vi "SVA 4MV6 T030 CCE RRMA .vi"() -> ()   [LabVIEW 2020]
doc: "Ceballos Conde Emanuel Rodríguez Ramírez Miguel Ángel 4MV6 Sistemas de visión artificial 2022/1\neste vi permite obtener el borde en escala de grises de una imagen asi como la malla conformada por el angulo phi de la imagen"
uses:
  <vilib>/Math Plots/3D Math Plots/3D Mesh/3D Mesh XCtrl/3D Mesh.xctl
  <vilib>/Math Plots/3D Math Plots/3D Mesh/3D Mesh Datatype/Public/Plot Helper (Matrix).vi
  <vilib>/Math Plots/3D Math Plots/3D Mesh/3D Mesh Datatype/3D Mesh Datatype.lvclass
panel:
  in  "obtener borde":bool
  in  "stop":bool
  out "3D Mesh":refnum<class "3D Plot Datatype.lvclass">[](xcontrol)
  in  "amp borde":u8=1
  out "new picture 2":picture
  out "new picture":picture
  in  "sig":i32=2
  in  "T":i32=3
  in  "CAPA DE COLOR":T1(ring)=enum."RGB2GRAY MATLAB"
  in  "file":path
  # "Ceballos Conde Emanuel\nRodríguez Ramírez Miguel Ángel\n4MV6\nSistemas de visión artificial\n2022/1"
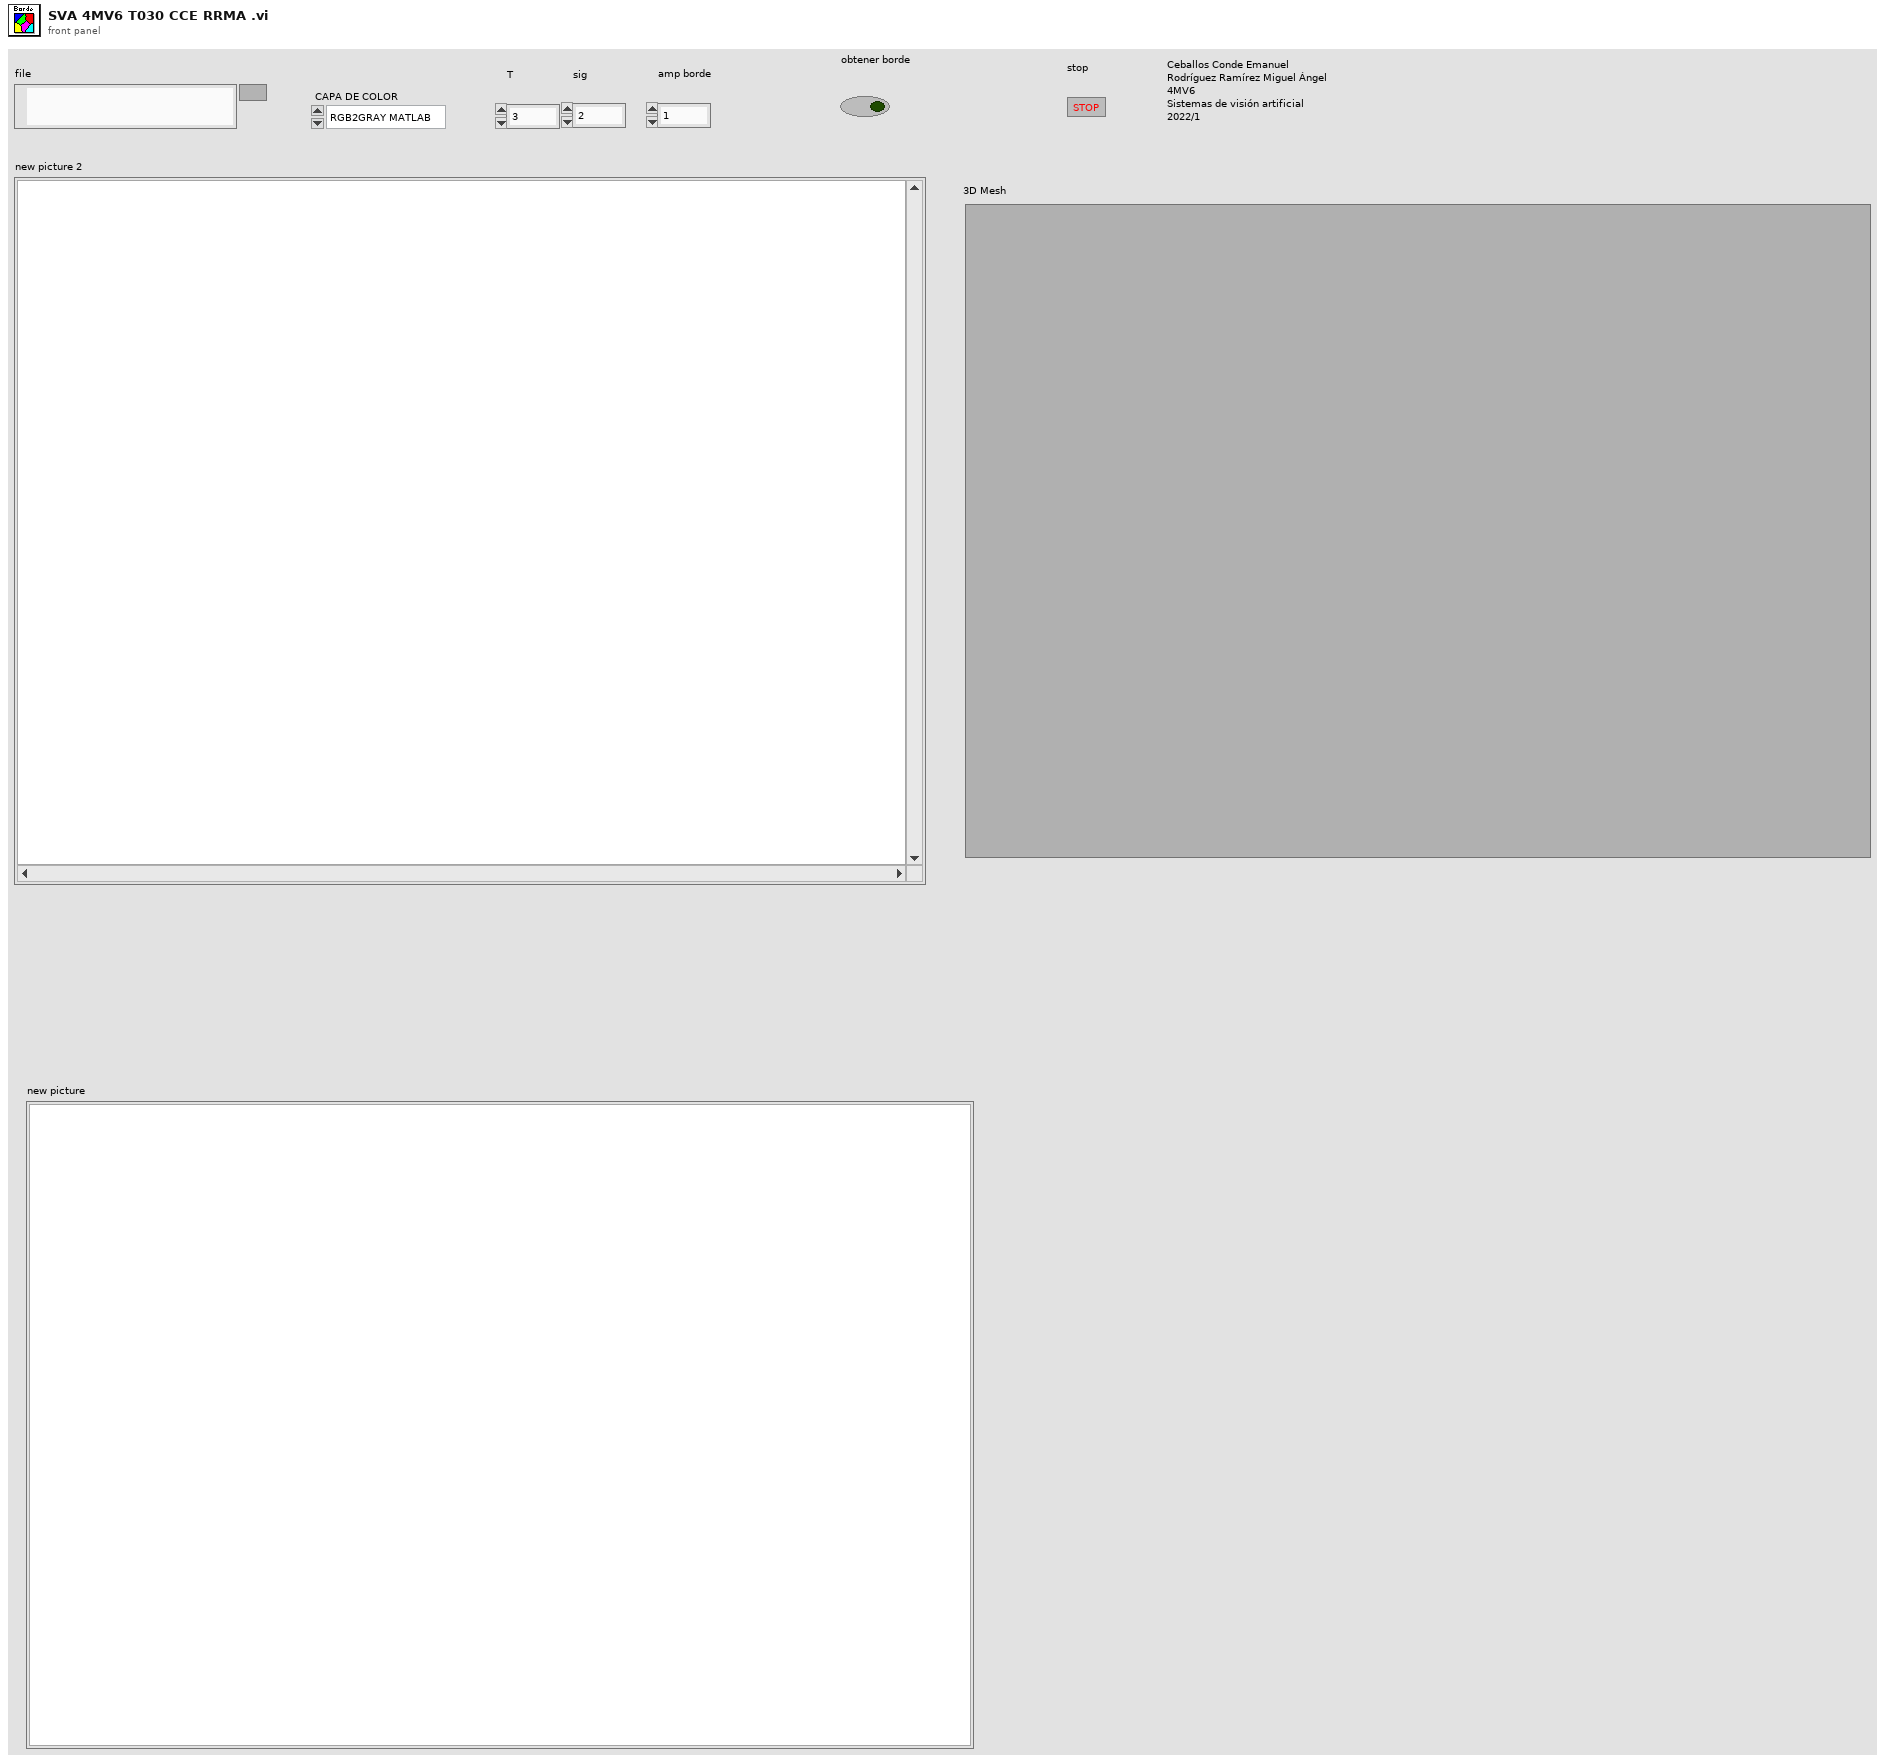
[diagram p1: front panel]
types:
  T1 = enum16{"H", "S", "V", "C", "M", "Y", "R", "G", "B", "RGB2GRAY MATLAB"}
  T2 = typedef "imagedata.ctl" = cluster{"image type":i32, "image depth":i32, "image":u8[], "mask":u8[], "colors":u32[], "Rectangle":cluster{"left":i16, "top":i16, "right":i16, "bottom":i16}}
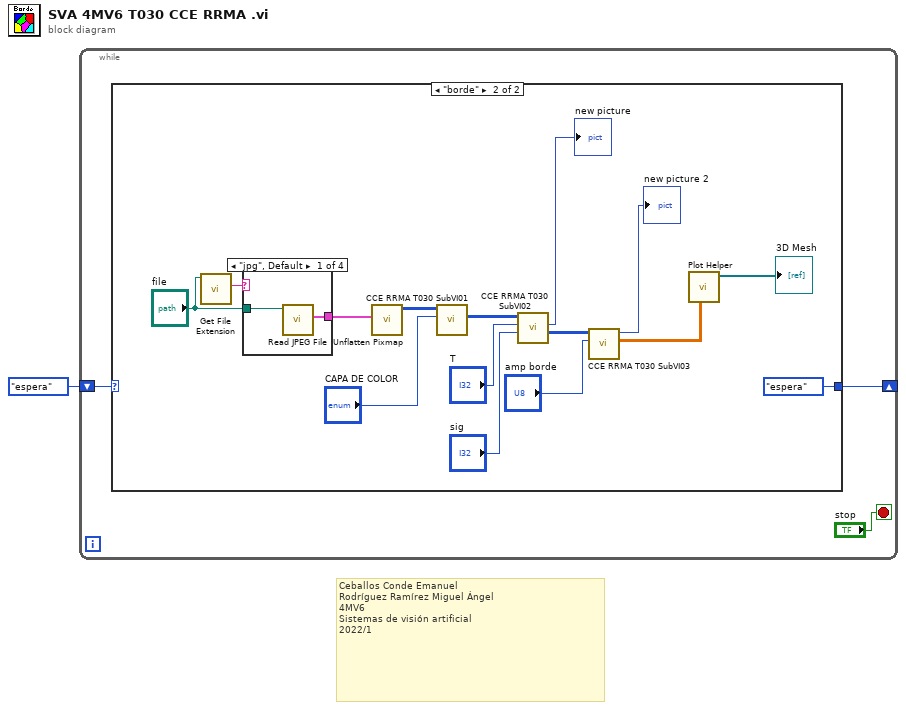
[diagram p0: block diagram]
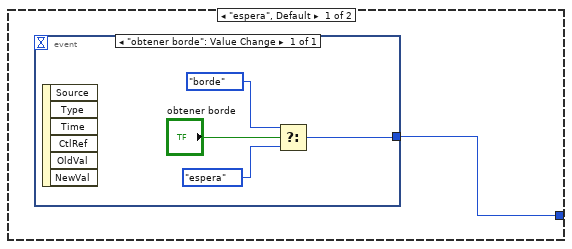
[diagram p2: hidden frame]
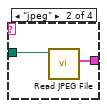
[diagram p3: hidden frame]
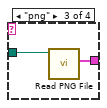
[diagram p4: hidden frame]
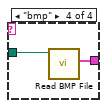
[diagram p5: hidden frame]
diagram:
  # "Ceballos Conde Emanuel\nRodríguez Ramírez Miguel Ángel\n4MV6\nSistemas de visión artificial\n2022/1"
  n1 = while {
    shift-right: [w2] -> _
    shift-left: enum16{"espera", "borde"}."espera" -> [w3]
    stop <- "stop" stop-if-true
    n2 = case shown="\"borde\"" w3 {
      tunnel: [w5 enum16{"espera", "borde"}."espera"] -> w2
      frame "espera", Default {
        n3 = event shown="[0] \"obtener borde\": Value Change" {
          selector: _ -> [_]
          dyn-events: _ -> [_]
          timeout: _ -> [_]
          tunnel: [w6] -> w5
          event "obtener borde": Value Change {
            n4 = event-data() -> ()  [unwired: 1 in, 6 out]
            n5 = Select(t=enum16{"espera", "borde"}."borde", s="obtener borde", f=enum16{"espera", "borde"}."espera") -> (s? t:f=w6:enum16{"espera", "borde"})
          }
        }
      }
      frame "borde" {
        n6 = call <vilib>:"Get File Extension.vi"("file"="file") -> ("lowercase file extension"=w24:string)  [unwired: 6 in, 4 out]
        n7 = case shown="\"jpg\", Default" w24 {
          tunnel: "file" -> [w26 w28 w30 w32]
          tunnel: [w25 w27 w29 w31] -> w23
          frame "jpg", Default {
            n8 = call <vilib>:"Read JPEG File.vi"("path to JPEG file"=w26) -> ("image data"=w25:T2)  [unwired: 8 in, 2 out]
          }
          frame "jpeg" {
            n9 = call <vilib>:"Read JPEG File.vi"("path to JPEG file"=w28) -> ("image data"=w27:T2)  [unwired: 8 in, 2 out]
          }
          frame "png" {
            n10 = call <vilib>:"Read PNG File.vi"("path to PNG file"=w30) -> ("image data"=w29:T2)  [unwired: 8 in, 2 out]
          }
          frame "bmp" {
            n11 = call <vilib>:"Read BMP File.vi"("path to BMP file"=w32) -> ("image data"=w31:T2)  [unwired: 8 in, 2 out]
          }
        }
        n12 = call <vilib>:"Unflatten Pixmap.vi"("image data"=w23) -> ("24-bit pixmap"=w19:u32[][])  [unwired: 4 in, 6 out]
        n13 = call "CCE RRMA T030 SubVI01.vi"("CAPA DE COLOR"="CAPA DE COLOR", "Image Pixels (U32)"=w19) -> ("capa u8"=w18:u8[][])  [unwired: 8 in, 1 out]
        n14 = call "CCE RRMA T030 SubVI02.vi"("sig"="sig", "T"="T", "capa"=w18) -> ("capa u8"=w17:u8[][], "new picture"=→"new picture":picture)  [unwired: 6 in, 1 out]
        n15 = call "CCE RRMA T030 SubVI03.vi"("amp borde"="amp borde", "capa u8"=w17) -> ("phi"=w13:sgl[][], "new picture"=→"new picture 2":picture)  [unwired: 8 in]
        n16 = call-poly <vilib>:"Plot Helper.vi"("z matrix"=w13) -> ("3D Plot lvclass Array out"=→"3D Mesh":refnum<class "3D Plot Datatype.lvclass">[])  [unwired: 5 in, 5 out]
      }
    }
  }
